vi "GetQueue.vi"(8 "error in (no error)":errorcluster caption="Fehler (Eingang, kein Fehler)", 11 "PassDataAround Eingang":refnum<class "PassDataAround.lvclass"> caption="DNL_LabVIEW Object in") -> (0 "error out":errorcluster caption="Fehler (Ausgang)", 3 "PassDataAround Ausgang":refnum<class "PassDataAround.lvclass"> caption="DNL_LabVIEW Object out")   [LabVIEW 2013]
uses:
  PassDataAround.lvclass
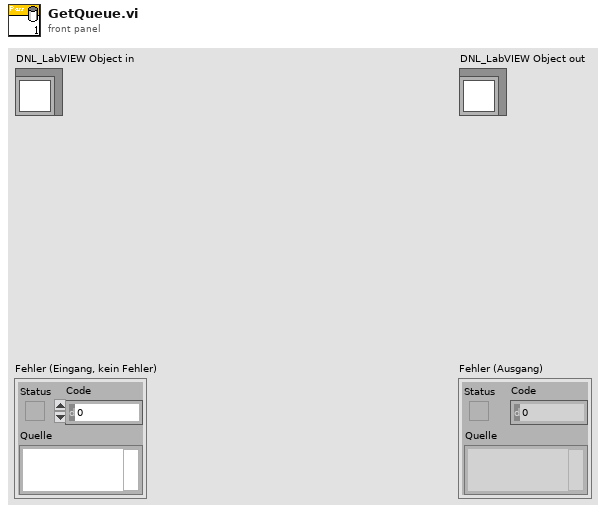
[diagram p1: front panel]
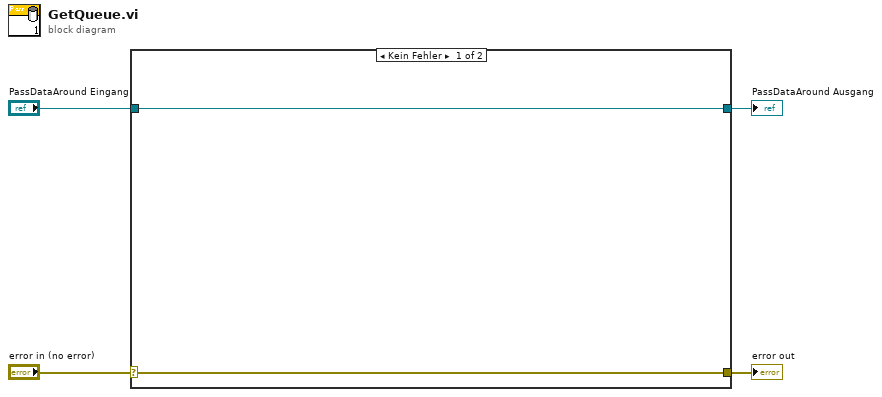
[diagram p0: block diagram]
diagram:
  n1 = case shown="Kein Fehler" "error in (no error)" {
    selector: "error in (no error)" -> [w5 w8]
    tunnel: [w5 w8] -> w3
    tunnel: [w6 w7] -> w1
    tunnel: "PassDataAround Eingang" -> [w6 w7]
    frame No Error {
    }
    frame Error {
    }
  }
  "error out" <- w3
  "PassDataAround Ausgang" <- w1
